vi "Constants.vi"() -> ()   [LabVIEW 2020, in "Communication Bus Template Scripting.lvlib"]
doc: "Use this Global VI to access the GUIDs assigned to the page resources of the Custom Device."
uses:
  Communication Bus Template Scripting.lvlib
panel:
  in  "Tab Control":enum32{"GUIDs", "Constants", "Properties"}(tab)=enum."Constants"
  in  "GUID.Disabled Custom Device":string="AB0B60A5-F604-4C3C-A8E4-523624E8891D"
  in  "GUID.Channel":string="0675c943-5444-47d6-a732-30e8170ca818"
  in  "GUID.Import Frames":string="db43d6e5-53fb-4f66-935d-3df211fac2b0"
  in  "GUID.Outgoing":string="4a2a8cff-0efe-4d8d-9297-6d7b1461b132"
  in  "GUID.Incoming":string="0806d046-d172-41c6-923a-ea2f0a033aaf"
  in  "GUID.Database":string="93c42860-b6b1-49e2-82f1-7f71f23907bd"
  in  "GUID.Add Database":string="cdc240f6-8a8e-4b98-b947-dc43e26f33eb"
  in  "GUID.Port":string="c33f961b-5445-4ca2-95c0-8ffbb92313cb"
  in  "GUID.Add Port":string="61f3d1e1-96da-4953-b846-b1921f4633dd"
  in  "GUID.Databases":string="0ea00ee9-bf24-4f89-bc82-a2a280190e7b"
  in  "GUID.Ports":string="54d3c231-5bbc-41bd-84f0-cbf6c48b59d0"
  in  "Protocol":string="936f3d3d-57f9-4ae0-ac61-b0abf738573d"
  in  "Vendor":string="350f1f90-dede-4c86-9a3d-8bedbf3ddc34"
  in  "GUID.Frame":string="12b029fd-7aaa-4aa7-9f3a-279e0ce107c0"
  in  "GUID.Custom Device":string="6d83d852-1383-4c81-9895-38ca2655dae3"
  in  "Channel":string="Channel"
  in  "Import Frames":string="Import Frames"
  in  "Frame":string="Frame"
  in  "Outgoing":string="Outgoing"
  in  "Incoming":string="Incoming"
  in  "Add Database":string="Add Database"
  in  "Database":string="Database"
  in  "Port":string="Port"
  in  "Add Port":string="Add Port"
  in  "Databases":string="Databases"
  in  "Ports":string="Ports"
  in  "Baud.Rate":string="Baud.Rate"
  in  "Database.Path":string="Database.Path"
  in  "Database.Name":string="Database.Name"
  in  "Frame.ID":string="Frame.ID"
  in  "Compiled.Settings":string="Compiled.Settings"
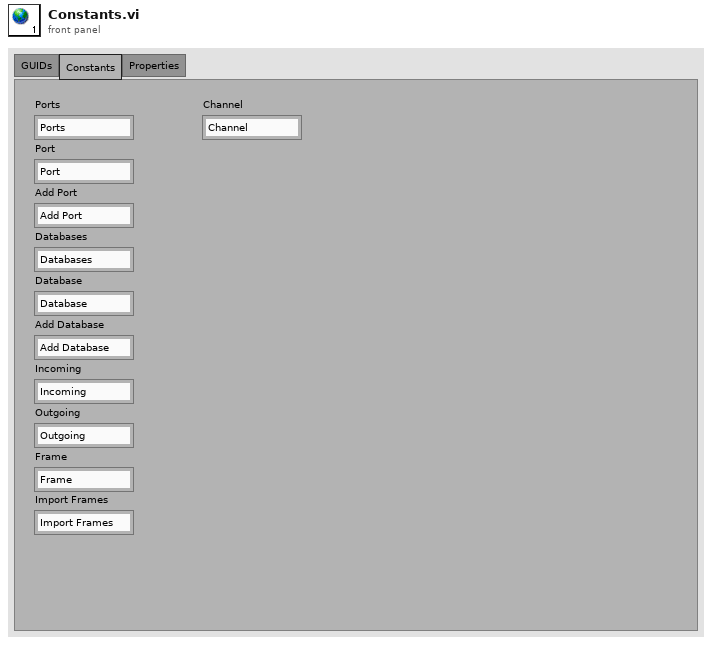
[diagram p1: front panel]
diagram:
